vi "UART.vi"() -> ()   [LabVIEW 2019]
uses:
  <vilib>/myRIO/Instrument Drivers/Onboard IO/UART/typedef/VISA Configuration.ctl
  <vilib>/Instr/_visa.llb/VISA Configure Serial Port (Instr).vi
  <vilib>/myRIO/Express VI/Onboard IO/UART/UART Express VI.xnode
  <vilib>/myRIO/Instrument Drivers/Onboard IO/UART/UART.lvlib
panel:
  out "Sensor 5":dbl
  out "Sensor 4":dbl
  out "Sensor_3":dbl
  out "Sensor_1":dbl
  out "Sensor_2":dbl
  out "Trama Recibida":string
  in  "Señal 5":dbl
  in  "Señal 4":dbl
  in  "Señal_3":dbl
  in  "Señal_2":dbl
  in  "Señal_1":dbl
  out "Trama de envio A":string
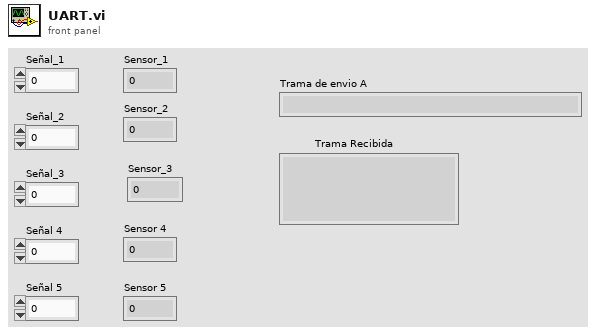
[diagram p1: front panel]
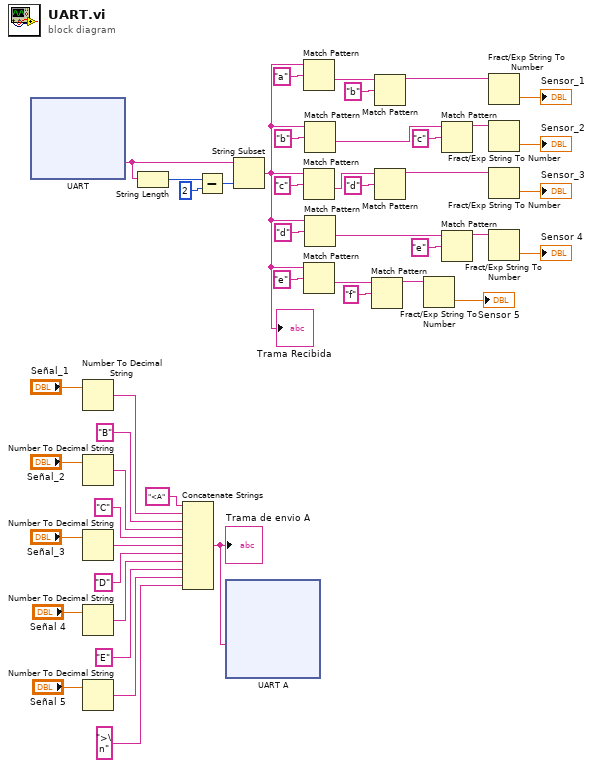
[diagram p0: block diagram]
diagram:
  n1 = xnode "UART"() -> ("Characters Read"=w1:string)  [unwired: 1 in, 1 out]
  n2 = Number To Decimal String(number="Señal_1") -> (decimal integer string=w31:string)  [unwired: 1 in]
  n3 = Number To Decimal String(number="Señal_2") -> (decimal integer string=w33:string)  [unwired: 1 in]
  n4 = Number To Decimal String(number="Señal_3") -> (decimal integer string=w35:string)  [unwired: 1 in]
  n5 = Number To Decimal String(number="Señal 4") -> (decimal integer string=w44:string)  [unwired: 1 in]
  n6 = Number To Decimal String(number="Señal 5") -> (decimal integer string=w46:string)  [unwired: 1 in]
  n7 = String Length(string=w1) -> (length=w3:i32)
  n8 = Concatenate Strings("<A" ("string"), w31, "B" ("string"), w33, "C" ("string"), w35, "D" ("string"), w44, "E" ("string"), w46, ">\n" ("string")) -> (w40:string)
  "Trama de envio A" <- w40
  n9 = Subtract(x=w3, y=2) -> (x-y=w5:i32)
  n10 = xnode "UART A"("Characters to Write"=w40) -> ()  [unwired: 1 in, 2 out]
  n11 = String Subset(string=w1, length (rest)=w5) -> (substring=w2:string)  [unwired: 1 in]
  "Trama Recibida" <- w2
  n12 = Match Pattern(string=w2, regular expression="a") -> (after substring=w30:string)  [unwired: 1 in, 3 out]
  n13 = Match Pattern(string=w2, regular expression="c") -> (after substring=w20:string)  [unwired: 1 in, 3 out]
  n14 = Match Pattern(string=w2, regular expression="e") -> (after substring=w10:string)  [unwired: 1 in, 3 out]
  n15 = Match Pattern(string=w2, regular expression="b") -> (after substring=w22:string)  [unwired: 1 in, 3 out]
  n16 = Match Pattern(string=w2, regular expression="d") -> (after substring=w12:string)  [unwired: 1 in, 3 out]
  n17 = Match Pattern(string=w10, regular expression="f") -> (before substring=w7:string)  [unwired: 1 in, 3 out]
  n18 = Match Pattern(string=w30, regular expression="b") -> (before substring=w26:string)  [unwired: 1 in, 3 out]
  n19 = Match Pattern(string=w20, regular expression="d") -> (before substring=w17:string)  [unwired: 1 in, 3 out]
  n20 = Fract/Exp String To Number(string=w7) -> (number=→"Sensor 5":dbl)  [unwired: 3 in, 1 out]
  n21 = Match Pattern(string=w22, regular expression="c") -> (before substring=w25:string)  [unwired: 1 in, 3 out]
  n22 = Match Pattern(string=w12, regular expression="e") -> (before substring=w15:string)  [unwired: 1 in, 3 out]
  n23 = Fract/Exp String To Number(string=w26) -> (number=→"Sensor_1":dbl)  [unwired: 3 in, 1 out]
  n24 = Fract/Exp String To Number(string=w25) -> (number=→"Sensor_2":dbl)  [unwired: 3 in, 1 out]
  n25 = Fract/Exp String To Number(string=w17) -> (number=→"Sensor_3":dbl)  [unwired: 3 in, 1 out]
  n26 = Fract/Exp String To Number(string=w15) -> (number=→"Sensor 4":dbl)  [unwired: 3 in, 1 out]
